vi "Xml_Save_Voltages.vi"(8 "error in (no error)":errorcluster, 11 "Refnum Clust":refnum<vi>) -> (0 "error out":errorcluster, 3 "XML String Out":string)   [LabVIEW 2020]
uses:
  controls/VOLTAGES_Inputs.ctl
  controls/HEXA_Inputs.ctl
  controls/QUAD_Inputs.ctl
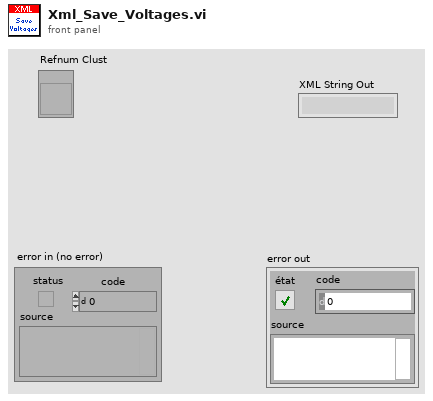
[diagram p1: front panel]
types:
  T1 = typedef "VOLTAGES_Inputs.ctl" = cluster{"Hexa 1":T2, "Hexa 2":T2, "Hexa 3":T2, "Quad 1":T3, "Quad 2":T3, "Quad 3":T3}
  T2 = typedef "HEXA_Inputs.ctl" = cluster{"Used":bool, "Voltage":dbl}
  T3 = typedef "QUAD_Inputs.ctl" = cluster{"Used":bool, "Voltage":dbl}
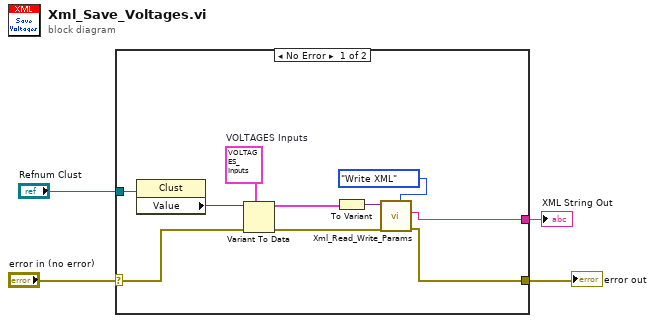
[diagram p0: block diagram]
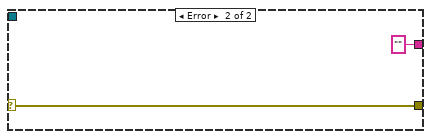
[diagram p2: hidden frame]
diagram:
  n1 = case shown="No Error" "error in (no error)" {
    selector: "error in (no error)" -> [w14 w16]
    tunnel: [w13 w16] -> w3
    tunnel: [w12 "" ("XML String Out")] -> w2
    tunnel: "Refnum Clust" -> [w6 _]
    frame No Error {
      w7 = T1 {"Hexa 1"={"Used"=TRUE, "Voltage"=25.0}, "Hexa 2"={"Used"=TRUE, "Voltage"=25.0}, "Hexa 3"={"Used"=TRUE, "Voltage"=25.0}, "Quad 1"={"Used"=TRUE, "Voltage"=25.0}, "Quad 2"={"Used"=TRUE, "Voltage"=25.0}, "Quad 3"={"Used"=TRUE, "Voltage"=25.0}}  # VOLTAGES Inputs
      n2 = property class="Clust"(reference=w6) -> ("Value"=w5:variant)  [unwired: 1 in, 2 out]
      n3 = Variant To Data(error in=w14, type=w7, Variant=w5) -> (data=w9:T1, error out=w8:errorcluster)
      n4 = To Variant(anything=w9) -> (Variant=w11:variant)
      n5 = call "Xml_Read_Write_Params.vi"("Variant"=w11, "error in (no error)"=w8, "Command"=enum16{"Read XML", "Set", "Get", "Write XML"}."Write XML") -> ("XML String Out"=w12:string, "error out"=w13:errorcluster)  [unwired: 4 in, 1 out]
    }
    frame Error {
    }
  }
  "error out" <- w3
  "XML String Out" <- w2
